vi "test Error Propagation.vi"(8 "error in":errorcluster, 11 "TestCase in":refnum<class "Scripting.lvclass">) -> (0 "error out":errorcluster, 3 "TestCase out":refnum<class "Scripting.lvclass">)   [LabVIEW 2020, in "Scripting.lvclass"]
uses:
  Scripting.lvclass
  C:/dev/git/niveristand-custom-device-testing-tools/VeriStandScriptingTestCase/VeriStandScriptingTestCase.lvclass
  niveristand-custom-device-testing-tools/VeriStandScriptingTestCase/VeriStandScriptingTestCase.lvclass/VeriStandScriptingTestCase.ctl
  <vilib>/NI VeriStand/Custom Device API/Custom Device Item Ref.ctl
  Shared/Address.ctl
  Shared/Terminal Endpoint.ctl
  Shared/Message Definition.ctl
  Shared/Message Type.ctl
  Shared/Parameter Definition.ctl
  niveristand-custom-device-testing-tools/VeriStandScriptingTestCase/Read Target.vi
  NationalInstruments.VeriStand.SystemDefinitionAPI
  <vilib>/addons/_JKI Toolkits/VI Tester/TestCase.llb/TestCase.lvclass
  Scripting/AIM MIL-STD-1553 Scripting.lvlib
  <vilib>/NI VeriStand/Custom Device API/Custom Device API.lvlib
  Shared/Acyclic Frame Definition.ctl
  C:/Program Files (x86)/National Instruments/LabVIEW 2020/vi.lib/addons/_JKI Toolkits/VI Tester/TestCase.llb/TestCase.lvclass
  C:/dev/git/niveristand-aim-milStd1553-custom-device/Source/Custom Device Support/Tests/Unit/Scripting/Scripting.lvclass
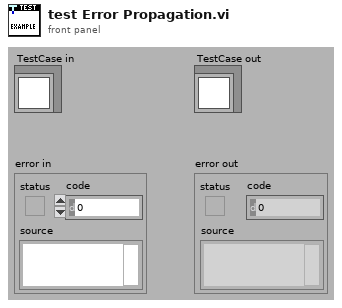
[diagram p1: front panel]
types:
  T1 = typedef "Custom Device API.lvlib/Custom Device Item Ref.ctl" = u64
  T2 = typedef "Acyclic Frame Definition.ctl" = cluster{"name":string, "messages":string[]}
  T3 = typedef "Message Definition.ctl" = cluster{"name":string, "message type":T4, "endpoint Tx":T5, "endpoint Rx":T5, "create timestamp channel":bool, "mode code":u16, "number of words":u16, "parameters":cluster{"name":string, "default value":dbl, "unit":string, "parameter definition":T7}[]}
  T4 = typedef "Message Type.ctl" = string
  T5 = typedef "Terminal Endpoint.ctl" = cluster{"terminal address":T6, "subaddress":T6}
  T6 = typedef "Address.ctl" = u16
  T7 = typedef "Parameter Definition.ctl" = cluster{"start index":i32, "size (bits)":i32, "encoding":enum16{"BNR", "BCD", "Discrete"}, "signed":bool, "multiplier":dbl, "offset":dbl}
  T8 = cluster{"Rx remote terminal":T5, "Rx remote terminal":T5}
  T9 = typedef "AIM Hardware Parameters.ctl" = cluster{"initialization method":T10, "card number":i32, "pxi slot number":i32, "biu number":i32, "bus selection":T11, "coupling mode":T12}
  T10 = typedef "Initialization Method.ctl" = enum16{"PXI Slot Number", "Card Number"}
  T11 = typedef "Bus Selection.ctl" = enum16{"Both", "Primary", "Secondary"}
  T12 = typedef "Coupling Mode.ctl" = enum16{"Isolated Onboard Termination", "Transformer Coupled", "Direct Coupled", "External with Onboard Termination", "Onboard Digital Wrap-around"}
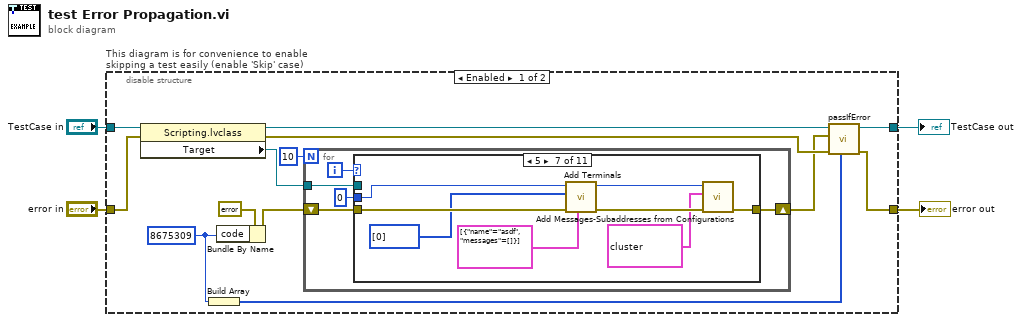
[diagram p0: block diagram]
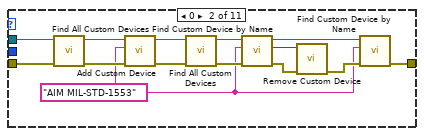
[diagram p3: hidden frame]
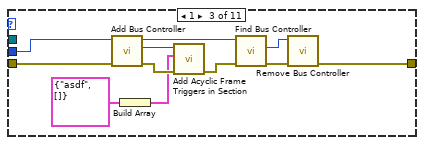
[diagram p4: hidden frame]
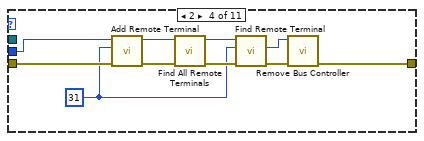
[diagram p5: hidden frame]
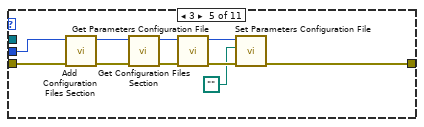
[diagram p6: hidden frame]
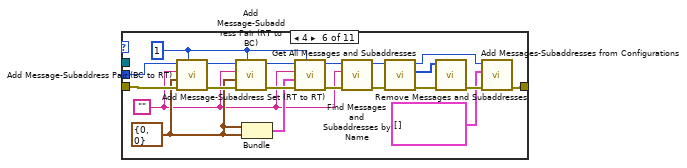
[diagram p7: hidden frame]
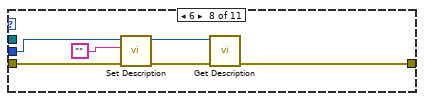
[diagram p8: hidden frame]
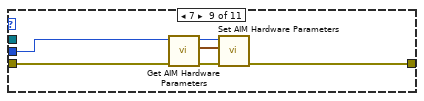
[diagram p9: hidden frame]
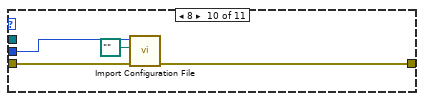
[diagram p10: hidden frame]
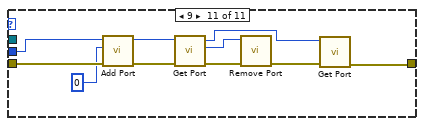
[diagram p11: hidden frame]
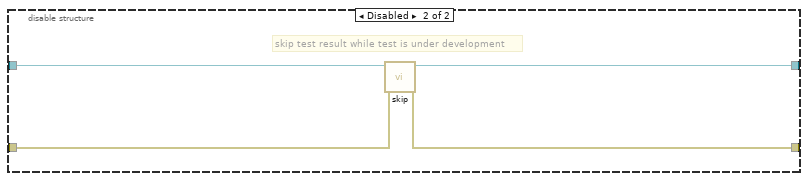
[diagram p12: hidden frame]
diagram:
  n1 = disable-structure "This diagram is for convenience to enable skipping a test easily (enable 'Skip' case)" shown="Enabled" {
    disable-tunnel: "TestCase in" -> [w15 w126]
    disable-tunnel: [w17 w124] -> w1
    disable-tunnel: [w16 w125] -> w3
    disable-tunnel: "error in" -> [w12 w123]
    frame Enabled {
      w8 = 8675309 ("code")
      n2 = property class="Scripting.lvclass"(reference=w15, error in=w12) -> (reference out=w14:refnum<class "Scripting.lvclass">, error out=w11:errorcluster, "Target"=w13:refnum<k24>)
      n3 = Build Array(w8) -> (w7:i32[])
      n4 = Bundle By Name(cluster=errorcluster {"status"=TRUE, "code"=-9999, "source"=""} ("error in"), "code"=w8) -> (w9:errorcluster)
      n5 = for {
        N: 10 -> [_]
        tunnel: w13 -> [w22]
        shift-right: [w20] -> w6
        shift-left: w9 -> [w21]
        i -> [w19]
        n6 = case shown="5" w19 {
          tunnel: w22 -> [_ w26 _ _ _ _ _ _ _ _ _]
          tunnel: w21 -> [w23 w25 w48 w58 w68 w79 w94 w102 w104 w111 w122]
          tunnel: [w23 w24 w46 w54 w62 w71 w95 w98 w103 w110 w114] -> w20
          tunnel: T1 0 ("Ballard MIL-STD 1553 custom device in") -> [_ _ w40 w49 w59 w73 w90 w101 w105 w112 w121]
          frame Default {
          }
          frame 0 {
            w28 = "AIM MIL-STD-1553" ("name")
            n7 = call "Find All Custom Devices.vi"("error in"=w25, "target"=w26) -> ("error out"=w37:errorcluster, "target out"=w36:refnum<k24>)  [unwired: 7 in, 1 out]
            n8 = call "Add Custom Device.vi"("error in"=w37, "custom device name"=w28, "target"=w36) -> ("error out"=w35:errorcluster, "target out"=w34:refnum<k24>)  [unwired: 6 in, 1 out]
            n9 = call "Find All Custom Devices.vi"("error in"=w35, "target"=w34) -> ("error out"=w33:errorcluster, "target out"=w32:refnum<k24>)  [unwired: 7 in, 1 out]
            n10 = call "Find Custom Device by Name.vi"("error in"=w33, "custom device name"=w28, "target"=w32) -> ("error out"=w31:errorcluster, "custom device"=w30:T1, "target out"=w27:refnum<k24>)  [unwired: 5 in, 1 out]
            n11 = call "Remove Custom Device.vi"("error in"=w31, "custom device ref"=w30) -> ("error out"=w29:errorcluster)  [unwired: 9 in]
            n12 = call "Find Custom Device by Name.vi"("error in"=w29, "custom device name"=w28, "target"=w27) -> ("error out"=w24:errorcluster)  [unwired: 5 in, 3 out]
          }
          frame 1 {
            n13 = call "Add Bus Controller.vi"("error in"=w48, "port"=w40) -> ("error out"=w42:errorcluster, "bus controller"=w43:T1, "port out"=w45:T1)  [unwired: 7 in]
            n14 = Build Array(T2 {"name"="asdf", "messages"=[]} ("acyclic frames")) -> (w38:T2[])
            n15 = call "Add Acyclic Frame Triggers in Section.vi"("error in"=w42, "acyclic frames"=w38, "acyclic frames section"=w43) -> ("error out"=w41:errorcluster)  [unwired: 7 in, 1 out]
            n16 = call "Find Bus Controller.vi"("error in"=w41, "port"=w45) -> ("error out"=w47:errorcluster, "bus controller"=w44:T1)  [unwired: 6 in, 2 out]
            n17 = call "Remove Bus Controller.vi"("error in"=w47, "bus controller"=w44) -> ("error out"=w46:errorcluster)  [unwired: 9 in]
          }
          frame 2 {
            w50 = T6 31 ("terminal address")
            n18 = call "Add Remote Terminal.vi"("error in"=w58, "terminal address"=w50, "port"=w49) -> ("error out"=w57:errorcluster, "port out"=w52:T1)  [unwired: 6 in, 1 out]
            n19 = call "Find All Remote Terminals.vi"("error in"=w57, "port"=w52) -> ("error out"=w56:errorcluster, "port out"=w51:T1)  [unwired: 7 in, 1 out]
            n20 = call "Find Remote Terminal.vi"("error in"=w56, "terminal address"=w50, "port"=w51) -> ("error out"=w55:errorcluster, "remote terminal"=w53:T1)  [unwired: 5 in, 2 out]
            n21 = call "Remove Bus Controller.vi"("error in"=w55, "bus controller"=w53) -> ("error out"=w54:errorcluster)  [unwired: 9 in]
          }
          frame 3 {
            n22 = call "Add Configuration Files Section.vi"("error in"=w68, "custom device"=w59) -> ("error out"=w67:errorcluster, "custom device out"=w65:T1)  [unwired: 7 in, 1 out]
            n23 = call "Get Configuration Files Section.vi"("error in"=w67, "custom device"=w65) -> ("error out"=w66:errorcluster, "custom device out"=w64:T1)  [unwired: 6 in, 2 out]
            n24 = call "Get Parameters Configuration File.vi"("error in"=w66, "custom device"=w64) -> ("error out"=w63:errorcluster, "custom device out"=w60:T1)  [unwired: 6 in, 2 out]
            n25 = call "Set Parameters Configuration File.vi"("error in"=w63, "parameters configuration file path"=path "", "custom device"=w60) -> ("error out"=w62:errorcluster)  [unwired: 7 in, 1 out]
          }
          frame 4 {
            w76 = T5 {"terminal address"=0, "subaddress"=0} ("Rx remote terminal")
            w74 = "" ("name")
            w77 = u16 1 ("number of words")
            n26 = call "Add Message-Subaddress Pair (BC to RT).vi"("number of words"=w77, "error in"=w79, "rx remote terminal"=w76, "name"=w74, "port"=w73) -> ("error out"=w87:errorcluster, "port out"=w88:T1)  [unwired: 3 in, 2 out]
            n27 = call "Add Message-Subaddress Pair (RT to BC).vi"("number of words"=w77, "error in"=w87, "tx remote terminal"=w76, "name"=w74, "port"=w88) -> ("error out"=w85:errorcluster, "port out"=w86:T1)  [unwired: 3 in, 2 out]
            n28 = Bundle("Rx remote terminal"=w76, "Rx remote terminal"=w76) -> (w75:T8)  [unwired: 1 in]
            n29 = call "Add Message-Subaddress Set (RT to RT).vi"("number of words"=w77, "error in"=w85, "remote terminals"=w75, "name"=w74, "port"=w86) -> ("error out"=w83:errorcluster, "port out"=w84:T1)  [unwired: 4 in, 1 out]
            n30 = call "Find Messages and Subaddresses by Name.vi"("error in"=w83, "name"=w74, "port"=w84) -> ("error out"=w81:errorcluster, "port out"=w82:T1)  [unwired: 5 in, 2 out]
            n31 = call "Get All Messages and Subaddresses.vi"("error in"=w81, "port"=w82) -> ("error out"=w80:errorcluster, "messages and subaddresses"=w78:T1[], "port out"=w70:T1)  [unwired: 7 in]
            n32 = call "Remove Messages and Subaddresses.vi"("error in"=w80, "messages or subaddresses"=w78) -> ("error out"=w72:errorcluster)  [unwired: 9 in]
            n33 = call "Add Messages-Subaddresses from Configurations.vi"("error in"=w72, "message configurations"=T3[] [] ("messages"), "port"=w70) -> ("error out"=w71:errorcluster)  [unwired: 7 in, 1 out]
          }
          frame 5 {
            n34 = call "Add Terminals.vi"("acyclic frames"=T2[] [{"name"="asdf", "messages"=[]}], "error in"=w94, "terminal addresses"=T6[] [0] ("terminals"), "port"=w90) -> ("error out"=w96:errorcluster, "port out"=w92:T1)  [unwired: 6 in]
            n35 = call "Add Messages-Subaddresses from Configurations.vi"("error in"=w96, "message configurations"=T3[] [{"name"="", "message type"="BC to RT", "endpoint Tx"={"terminal address"=0, "subaddress"=0}, "endpoint Rx"={"terminal address"=0, "subaddress"=0}, "create timestamp channel"=FALSE, "mode code"=0, "number of words"=0, "parameters"=[{"name"="p0", "default value"=1.0, "unit"="", "parameter definition"={"start index"=0, "size (bits)"=16, "encoding"=enum."BNR", "signed"=TRUE, "multiplier"=1.0, "offset"=0.0}}]}] ("messages"), "port"=w92) -> ("error out"=w95:errorcluster)  [unwired: 7 in, 1 out]
          }
          frame 6 {
            n36 = call "Set Description.vi"("error in"=w102, "description"="", "custom device"=w101) -> ("error out"=w100:errorcluster, "custom device out"=w99:T1)  [unwired: 7 in]
            n37 = call "Get Description.vi"("error in"=w100, "custom device"=w99) -> ("error out"=w98:errorcluster)  [unwired: 7 in, 2 out]
          }
          frame 7 {
            n38 = call "Get AIM Hardware Parameters.vi"("error in"=w104, "custom device"=w105) -> ("error out"=w107:errorcluster, "aim hardware parameters"=w106:T9, "custom device out"=w108:T1)  [unwired: 7 in]
            n39 = call "Set AIM Hardware Parameters.vi"("error in"=w107, "aim hardware parameters"=w106, "custom device"=w108) -> ("error out"=w103:errorcluster)  [unwired: 7 in, 1 out]
          }
          frame 8 {
            n40 = call "Import Configuration File.vi"("error in"=w111, "parameters configuration file path"=path "", "custom device"=w112) -> ("error out"=w110:errorcluster)  [unwired: 7 in, 1 out]
          }
          frame 9 {
            n41 = call "Add Port.vi"("error in"=w122, "port number"=u16 0, "custom device"=w121) -> ("error out"=w118:errorcluster, "custom device out"=w119:T1)  [unwired: 6 in, 1 out]
            n42 = call "Get Port.vi"("error in"=w118, "custom device ref"=w119) -> ("error out"=w117:errorcluster, "port"=w116:T1, "custom device ref out"=w113:T1)  [unwired: 6 in, 1 out]
            n43 = call "Remove Port.vi"("error in"=w117, "custom device ref"=w116) -> ("error out"=w115:errorcluster)  [unwired: 7 in, 2 out]
            n44 = call "Get Port.vi"("error in"=w115, "custom device ref"=w113) -> ("error out"=w114:errorcluster)  [unwired: 6 in, 3 out]
          }
        }
      }
      n45 = call-dynamic "passIfError.vi"("passing error codes (default = any error code)"=w7, "error in (no error)"=w11, "error"=w6, "TestCase in"=w14) -> ("error out"=w16:errorcluster, "TestCase out"=w17:refnum<class "Scripting.lvclass">)  [unwired: 6 in]
    }
    frame Disabled {
      # "skip test result while test is under development"
      n46 = call <vilib>:"skip.vi"("error in (no error)"=w123, "TestCase in"=w126) -> ("error out"=w125:errorcluster, "TestCase out"=w124:refnum<class "Scripting.lvclass">)  [unwired: 8 in]
    }
  }
  "error out" <- w3
  "TestCase out" <- w1
